vi "Configure Trigger (Transition).vi"(0 "VISA resource name":refnum<visa-resource-name>, 1 "Upper Level (1.2V)":dbl=1.2, 2 "Lower Level (-0.1V)":dbl=-0.1, 3 "Slope (0:Positive)":u16(ring) items=["Positive", "Negative", "Either"], 5 "Source (0:Channel1)":u16(ring) items=["Channel1", "Channel2", "Channel3", "Channel4", "Digital Channel0", "Digital Channel1", "Digital Channel2", "Digital Channel3", "Digital Channel4", "Digital Channel5", "Digital Channel6", "Digital Channel7", "Digital Channel8", "Digital Channel9", "Digital Channel10", "Digital Channel11", "Digital Channel12", "Digital Channel13", "Digital Channel14", "Digital Channel15"], 9 "Trigger Condition (0:Greater Than)":u16(ring) items=["Greater Than", "Less Than"], 11 "error in (no error)":errorcluster, 12 "Time (5E-10s)":dbl=5e-10, 13 "Trigger If Violation (0:Occurs)":u16(ring) items=["Occurs", "Logic"], 14 "Trigger Event (0:A Event)":u16(ring) items=["A Event", "B Event"]) -> (4 "VISA resource name out":refnum<visa-resource-name>, 6 "Trigger Event Out":u16(ring) items=["A Event", "B Event"], 15 "error out":errorcluster)   [LabVIEW 2011, in "Tektronix 7000 Series.lvlib"]
doc: "Configures transition trigger settings for an oscilloscope. A transition occurs when a pulse crosses both thresholds in the same direction as the specified polarity and the transition time between the two threshold crossings is greater or less than the specified time delta.\n\nTDS5000,TDS5000B,TDS6000,CSA7000 and TDS7000 series oscilloscopes don't support B Transition Trigger."
uses:
  Tektronix 7000 Series.lvlib
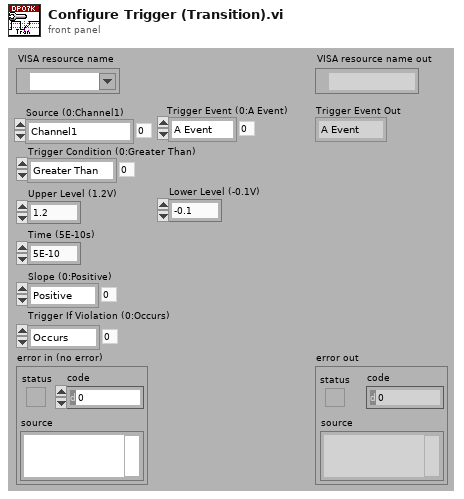
[diagram p1: front panel]
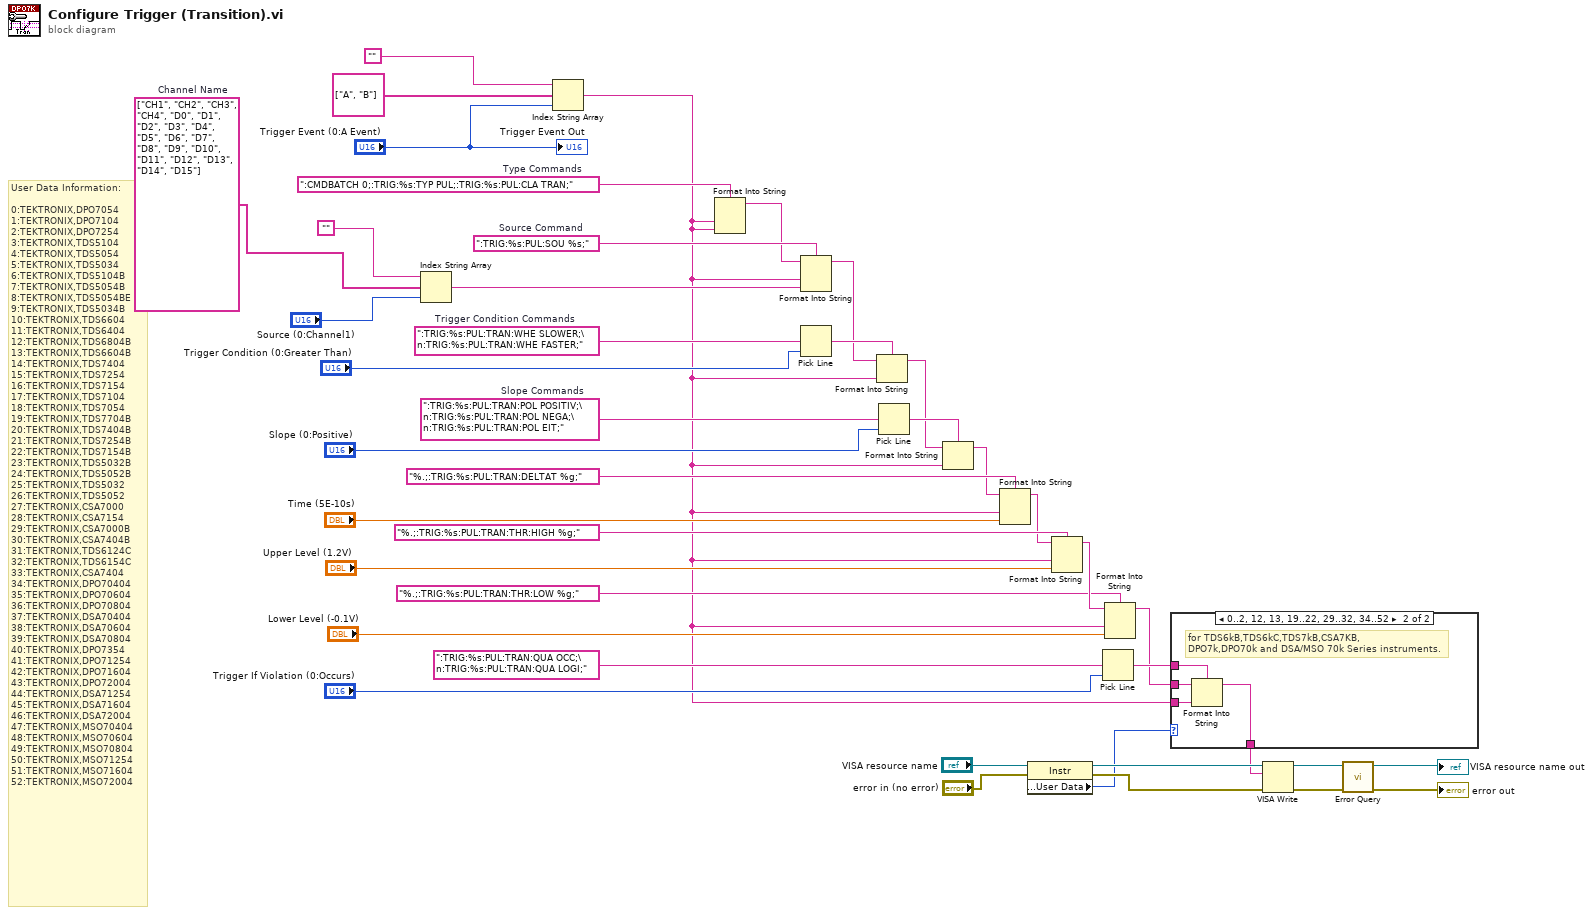
[diagram p0: block diagram]
diagram:
  w2 = string[] ["CH1", "CH2", "CH3", "CH4", "D0", "D1", "D2", "D3", "D4", "D5", "D6", "D7", "D8", "D9", "D10", "D11", "D12", "D13", "D14", "D15"]  # Channel Name
  w28 = ":TRIG:%s:PUL:TRAN:POL POSITIV;\n:TRIG:%s:PUL:TRAN:POL NEGA;\n:TRIG:%s:PUL:TRAN:POL EIT;"  # Slope Commands
  w30 = ":TRIG:%s:PUL:TRAN:WHE SLOWER;\n:TRIG:%s:PUL:TRAN:WHE FASTER;"  # Trigger Condition Commands
  w32 = ":TRIG:%s:PUL:SOU %s;"  # Source Command
  w23 = ":CMDBATCH 0;:TRIG:%s:TYP PUL;:TRIG:%s:PUL:CLA TRAN;"  # Type Commands
  # "User Data Information:\n\n0:TEKTRONIX,DPO7054\n1:TEKTRONIX,DPO7104\n2:TEKTRONIX,DPO7254\n3:TEKTRONIX,TDS5104\n4:TEKTRONIX,TDS5054\n5:TEKTRONIX,TDS5034\n6:TEKTRONIX,TDS5104B\n7:TEKTRONIX,TDS5054B\n8:TEKTRONIX,TDS5054BE\n9:TEKTRONIX,TDS5034B\n10:TEKTRONIX,TDS6604\n11:TEKTRONIX,TDS6404\n12:TEKTRONIX,TDS6804B\n13:TEKTRONIX,TDS6604B\n14:TEKTRONIX,TDS7404\n15:TEKTRONIX,TDS7254\n16:TEKTRONIX,TDS7154\n17:TEKTRONIX,TDS7104\n18:TEKTRONIX,TDS7054\n19:TEKTRONIX,TDS7704B\n20:TEKTRONIX,TDS7404B\n21:TEKTRONIX,TDS7254B\n22:TEKTRONIX,TDS7154B\n23:TEKTRONIX,TDS5032B\n24:TEKTRONIX,TDS5052B\n25:TEKTRONIX,TDS5032\n26:TEKTRONIX,TDS5052\n27:TEKTRONIX,CSA7000\n28:TEKTRONIX,CSA7154\n29:TEKTRONIX,CSA7000B\n30:TEKTRONIX,CSA7404B\n31:TEKTRONIX,TDS6124C\n32:TEKTRONIX,TDS6154C\n33:TEKTRONIX,CSA7404\n34:TEKTRONIX,DPO70404\n35:TEKTRONIX,DPO70604\n36:TEKTRONIX,DPO70804\n37:TEKTRONIX,DSA70404\n38:TEKTRONIX,DSA70604\n39:TEKTRONIX,DSA70804\n40:TEKTRONIX,DPO7354\n41:TEKTRONIX,DPO71254\n42:TEKTRONIX,DPO71604\n43:TEKTRONIX,DPO72004\n44:TEKTRONIX,DSA71254\n45:TEKTRONIX,DSA71604\n46:TEKTRONIX,DSA72004\n47:TEKTRONIX,MSO70404\n48:TEKTRONIX,MSO70604\n49:TEKTRONIX,MSO70804\n50:TEKTRONIX,MSO71254\n51:TEKTRONIX,MSO71604\n52:TEKTRONIX,MSO72004"
  n1 = Index String Array(1:"Source (0:Channel1)", 2:w2, 3:"" ("Empty String Constant")) -> (0:w22:string)
  n2 = Index String Array(1:"Trigger Event (0:A Event)", 2:string[] ["A", "B"], 3:"" ("Empty String Constant")) -> (0:w6:string)
  n3 = Format Into String(format string=w23, w6, w6) -> (resulting string=w12:string)  [unwired: 2 in, 1 out]
  n4 = Format Into String(format string=w32, initial string=w12, w6, w22) -> (resulting string=w20:string)  [unwired: 1 in, 1 out]
  n5 = Pick Line(multi-line string=w30, line index="Trigger Condition (0:Greater Than)") -> (output string=w21:string)  [unwired: 1 in]
  n6 = Format Into String(format string=w21, initial string=w20, w6) -> (resulting string=w17:string)  [unwired: 1 in, 1 out]
  n7 = Pick Line(multi-line string=w28, line index="Slope (0:Positive)") -> (output string=w18:string)  [unwired: 1 in]
  n8 = Format Into String(format string=w18, initial string=w17, w6) -> (resulting string=w11:string)  [unwired: 1 in, 1 out]
  n9 = Format Into String(format string="%.;:TRIG:%s:PUL:TRAN:DELTAT %g;", initial string=w11, w6, "Time (5E-10s)") -> (resulting string=w26:string)  [unwired: 1 in, 1 out]
  n10 = property class="Instr"(reference="VISA resource name", error in="error in (no error)") -> (reference out=w8:refnum<visa-resource-name>, error out=w7:errorcluster, "General Settings:User Data"=w4:u32)
  n11 = Format Into String(format string="%.;:TRIG:%s:PUL:TRAN:THR:HIGH %g;", initial string=w26, w6, "Upper Level (1.2V)") -> (resulting string=w25:string)  [unwired: 1 in, 1 out]
  n12 = Pick Line(multi-line string=":TRIG:%s:PUL:TRAN:QUA OCC;\n:TRIG:%s:PUL:TRAN:QUA LOGI;" ("Commands"), line index="Trigger If Violation (0:Occurs)") -> (output string=w16:string)  [unwired: 1 in]
  n13 = Format Into String(format string="%.;:TRIG:%s:PUL:TRAN:THR:LOW %g;", initial string=w25, w6, "Lower Level (-0.1V)") -> (resulting string=w5:string)  [unwired: 1 in, 1 out]
  n14 = case shown="0..2, 12, 13, 19..22, 29..32, 34..52" w4 {
    tunnel: w16 -> [_ w47]
    tunnel: w6 -> [_ w46]
    tunnel: w5 -> [w43 w45]
    tunnel: [w43 w44] -> w3
    frame Default {
    }
    frame 0..2, 12, 13, 19..22, 29..32, 34..52 {
      # "for TDS6kB,TDS6kC,TDS7kB,CSA7KB, \nDPO7k,DPO70k and DSA/MSO 70k Series instruments."
      n15 = Format Into String(format string=w47, initial string=w45, w46) -> (resulting string=w44:string)  [unwired: 1 in, 1 out]
    }
  }
  n16 = VISA Write(VISA resource name=w8, write buffer=w3, error in (no error)=w7) -> (VISA resource name out=w41:refnum<visa-resource-name>, error out=w42:errorcluster)  [unwired: 1 out]
  n17 = call "Error Query.vi"("error in (no error)"=w42, "VISA resource name"=w41) -> ("error out"=→"error out":errorcluster, "VISA resource name out"=→"VISA resource name out":refnum<visa-resource-name>)  [unwired: 6 in, 2 out]
  "Trigger Event Out" <- "Trigger Event (0:A Event)"
